vi "Editor Daten speichern (Sub.vi).vi"(0 "4":dbl[][](array[numeric]), 1 "Z 4":string, 2 "5":dbl[][](array[numeric]), 3 "Z 5":string, 4 "6":dbl[][](array[numeric]), 5 "Z 6":string, 6 "7":dbl[][](array[numeric]), 7 "Z 7":string, 8 "3":dbl[][](array[numeric]), 9 "8":dbl[][](array[numeric]), 10 "Z 3":string, 11 "Z 8":string, 12 "2":dbl[][](array[numeric]), 13 "9":dbl[][](array[numeric]), 14 "Z 2":string, 15 "Z 9":string, 16 "1":dbl[][](array[numeric]), 17 "10":dbl[][](array[numeric]), 18 "Z 1":string, 19 "Z 10":string, 21 "Formatierung+Namen":string="%d", 25 "Daten":string="%d", 26 "Modulname":string="%d") -> (23 "Ausgang":string)   [LabVIEW 2010]
panel:
  out "Verknüpfter String":string
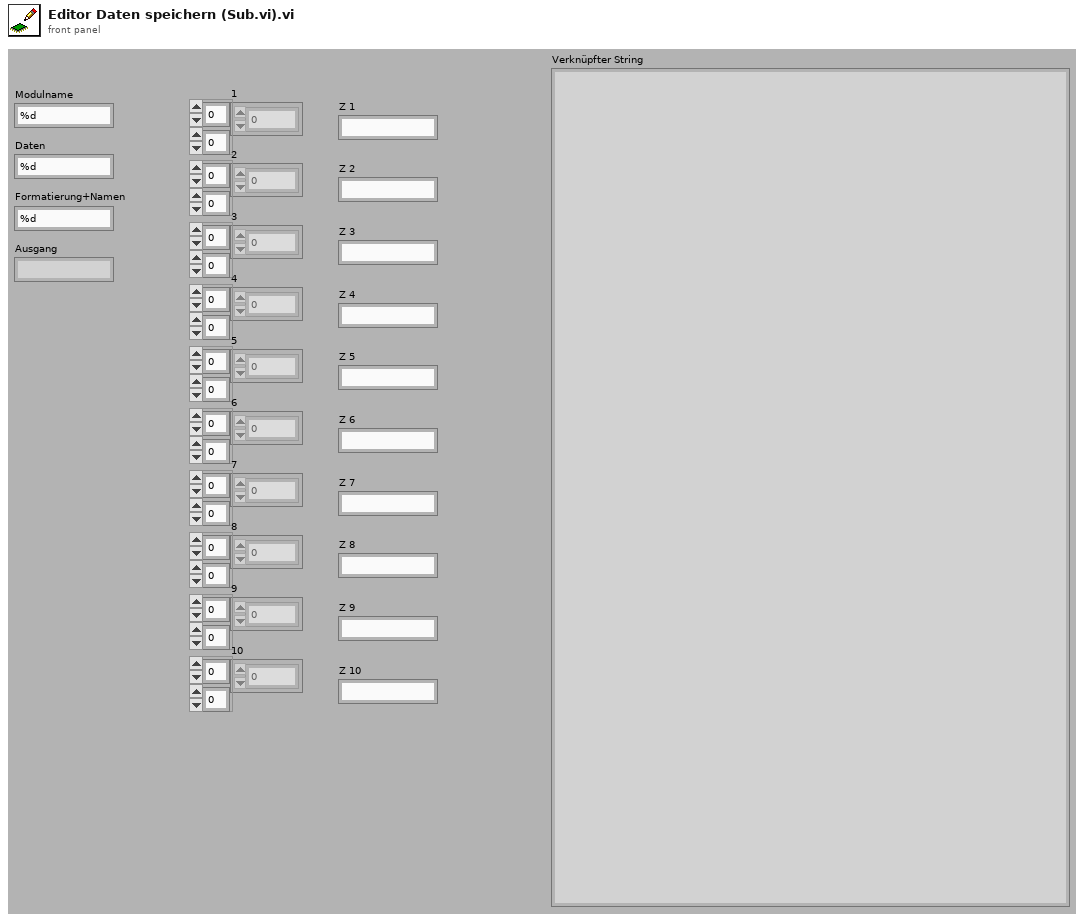
[diagram p1: front panel]
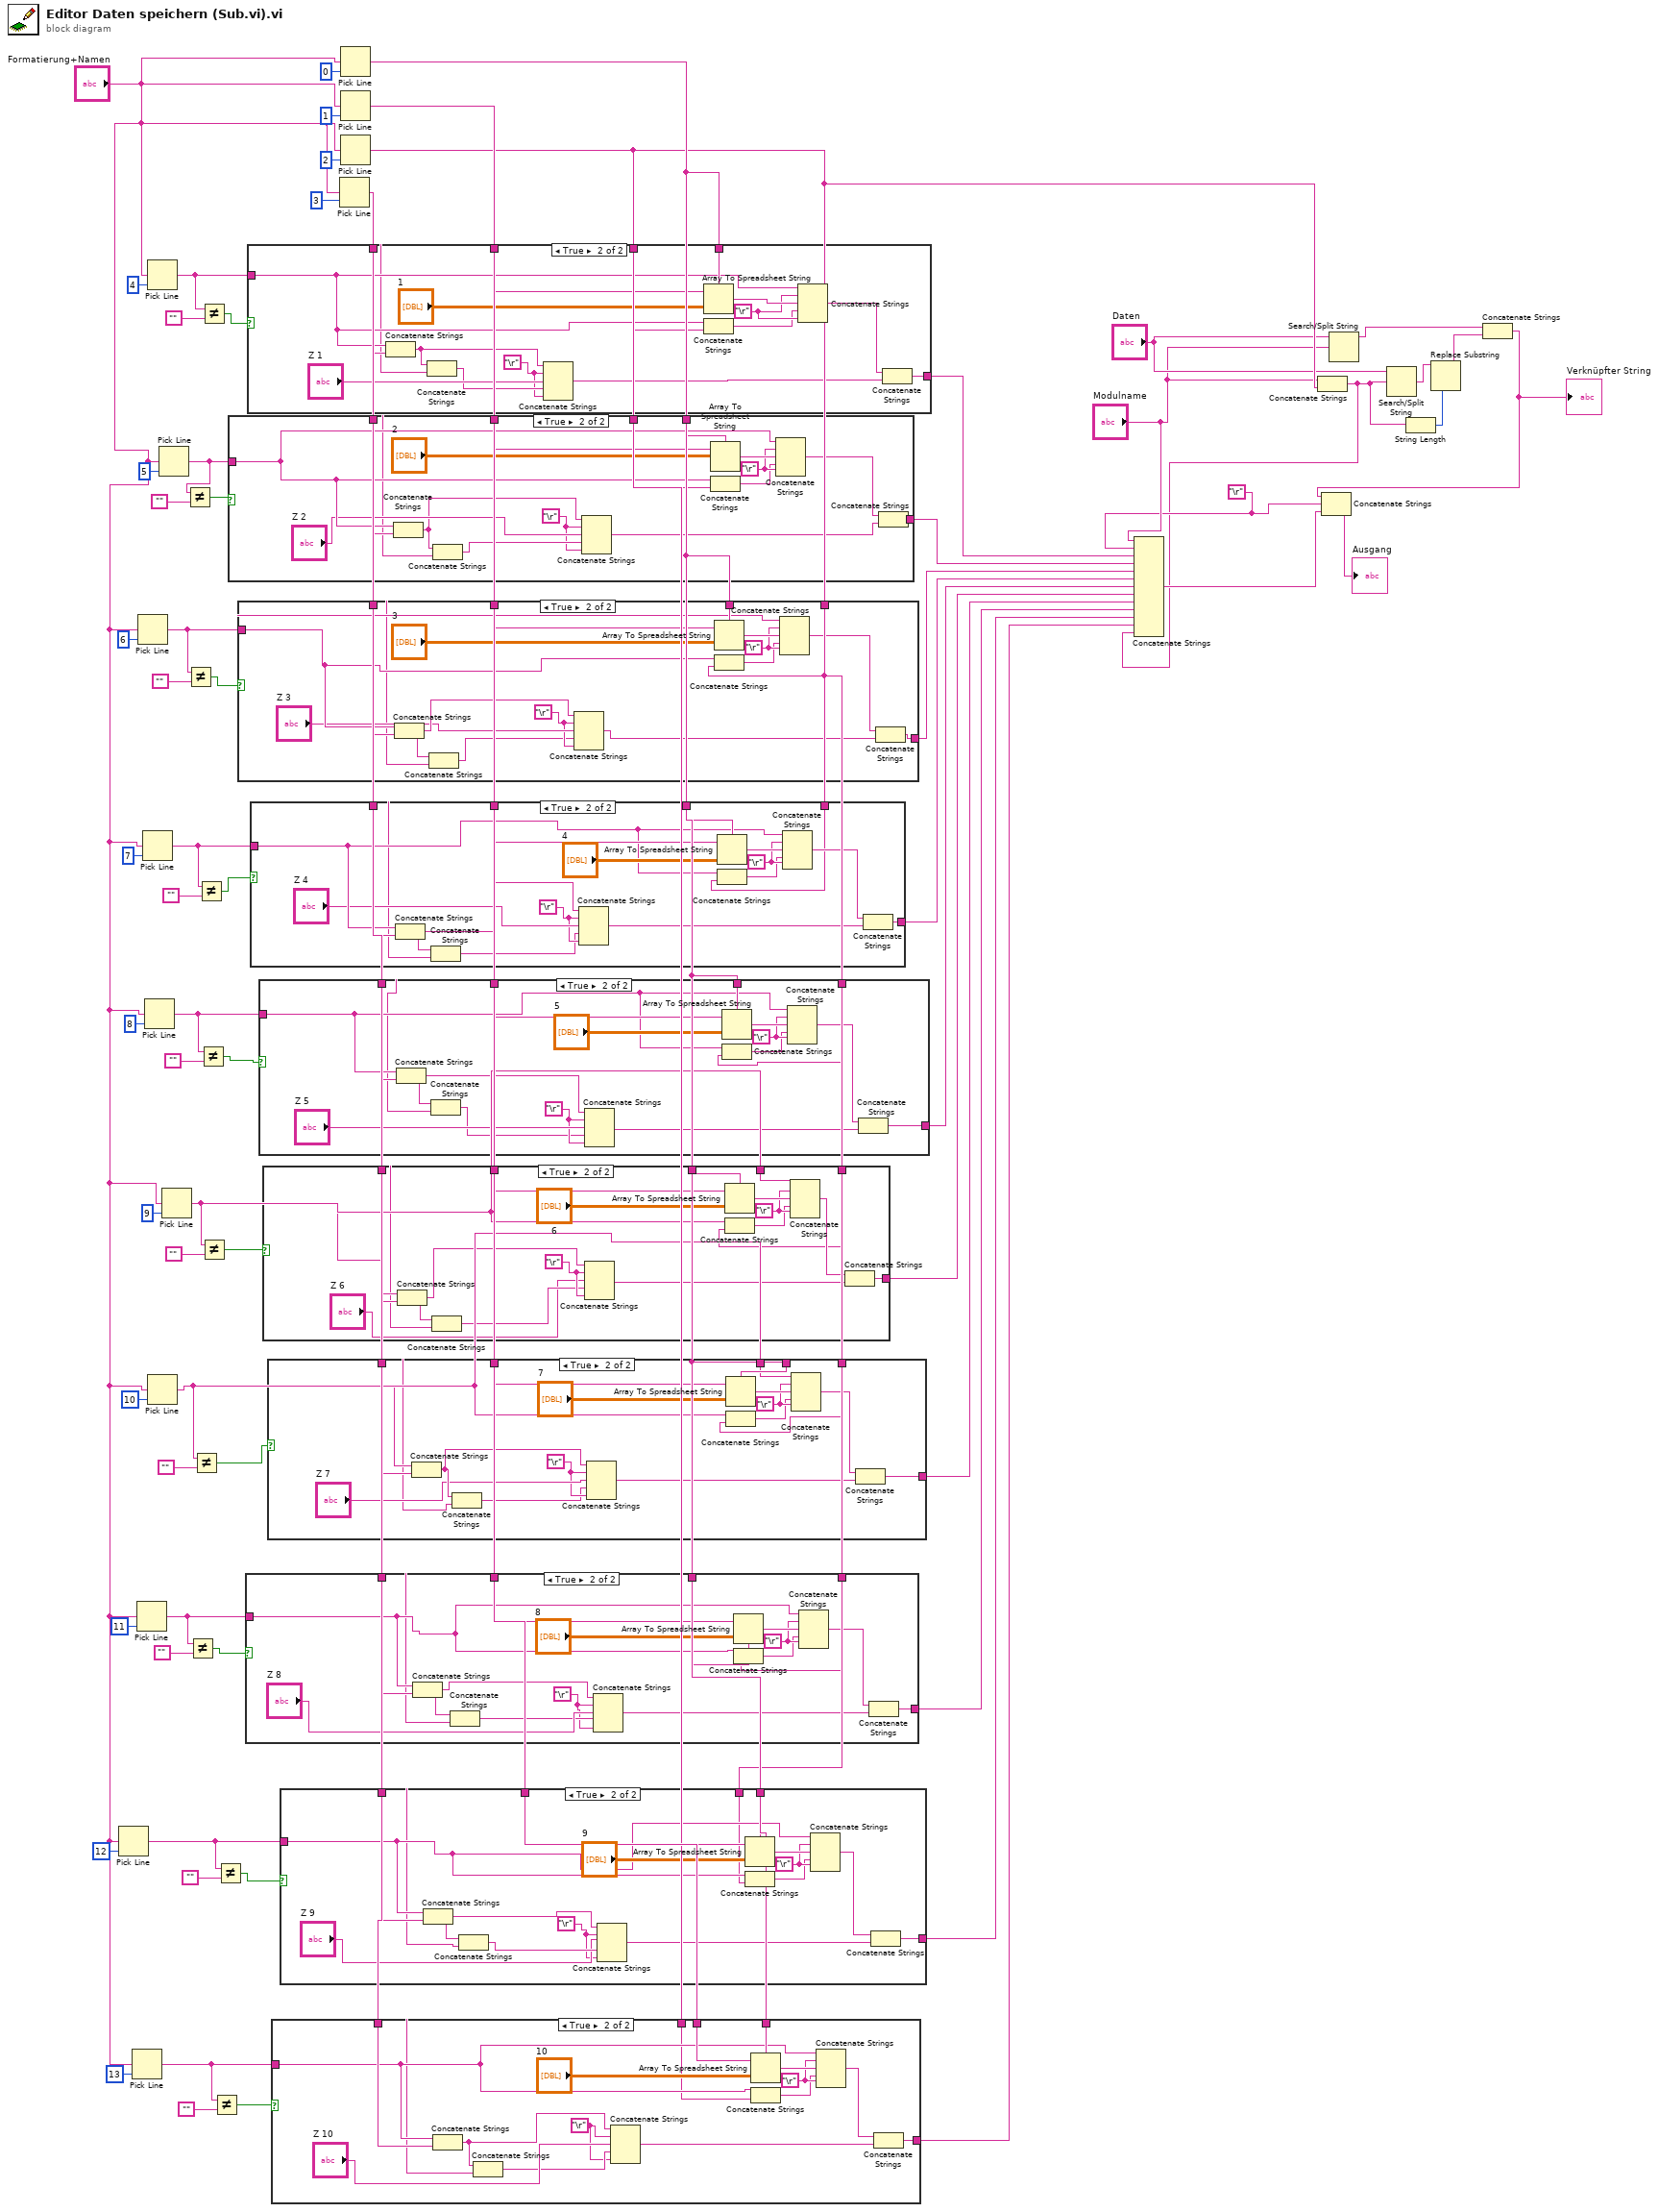
[diagram p0: block diagram]
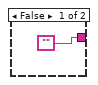
[diagram p2: hidden frame]
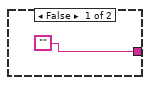
[diagram p3: hidden frame]
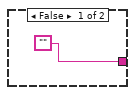
[diagram p4: hidden frame]
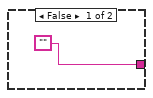
[diagram p5: hidden frame]
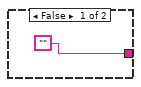
[diagram p6: hidden frame]
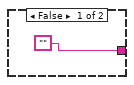
[diagram p7: hidden frame]
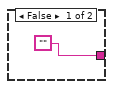
[diagram p8: hidden frame]
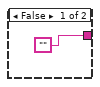
[diagram p9: hidden frame]
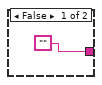
[diagram p10: hidden frame]
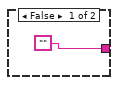
[diagram p11: hidden frame]
diagram:
  w32 = "\r"
  n1 = Pick Line(multi-line string="Formatierung+Namen", line index=12 ("Zeilenindex")) -> (output string=w15:string)  [unwired: 1 in]
  n2 = Pick Line(multi-line string="Formatierung+Namen", line index=13 ("Zeilenindex")) -> (output string=w17:string)  [unwired: 1 in]
  n3 = Pick Line(multi-line string="Formatierung+Namen", line index=11 ("Zeilenindex")) -> (output string=w13:string)  [unwired: 1 in]
  n4 = Pick Line(multi-line string="Formatierung+Namen", line index=6 ("Zeilenindex")) -> (output string=w3:string)  [unwired: 1 in]
  n5 = Pick Line(multi-line string="Formatierung+Namen", line index=7 ("Zeilenindex")) -> (output string=w6:string)  [unwired: 1 in]
  n6 = Pick Line(multi-line string="Formatierung+Namen", line index=8 ("Zeilenindex")) -> (output string=w7:string)  [unwired: 1 in]
  n7 = Pick Line(multi-line string="Formatierung+Namen", line index=4 ("Zeilenindex")) -> (output string=w29:string)  [unwired: 1 in]
  n8 = Pick Line(multi-line string="Formatierung+Namen", line index=10 ("Zeilenindex")) -> (output string=w11:string)  [unwired: 1 in]
  n9 = Pick Line(multi-line string="Formatierung+Namen", line index=5 ("Zeilenindex")) -> (output string=w1:string)  [unwired: 1 in]
  n10 = Pick Line(multi-line string="Formatierung+Namen", line index=9 ("Zeilenindex")) -> (output string=w9:string)  [unwired: 1 in]
  n11 = Not Equal?(x=w1, y="") -> (x != y?=w2:bool)
  n12 = Not Equal?(x=w3, y="") -> (x != y?=w4:bool)
  n13 = Not Equal?(x=w13, y="") -> (x != y?=w14:bool)
  n14 = Not Equal?(x=w11, y="") -> (x != y?=w12:bool)
  n15 = Not Equal?(x=w6, y="") -> (x != y?=w5:bool)
  n16 = Not Equal?(x=w7, y="") -> (x != y?=w8:bool)
  n17 = Not Equal?(x=w29, y="") -> (x != y?=w30:bool)
  n18 = Not Equal?(x=w9, y="") -> (x != y?=w10:bool)
  n19 = Not Equal?(x=w17, y="") -> (x != y?=w18:bool)
  n20 = Not Equal?(x=w15, y="") -> (x != y?=w16:bool)
  n21 = Pick Line(multi-line string="Formatierung+Namen", line index=3 ("Zeilenindex")) -> (output string=w53:string)  [unwired: 1 in]
  n22 = Pick Line(multi-line string="Formatierung+Namen", line index=0 ("Zeilenindex")) -> (output string=w66:string)  [unwired: 1 in]
  n23 = Pick Line(multi-line string="Formatierung+Namen", line index=1 ("Zeilenindex")) -> (output string=w67:string)  [unwired: 1 in]
  n24 = Pick Line(multi-line string="Formatierung+Namen", line index=2 ("Zeilenindex")) -> (output string=w42:string)  [unwired: 1 in]
  n25 = case shown="True" w2 {
    tunnel: w67 -> [_ w83]
    tunnel: w66 -> [_ w82]
    tunnel: w53 -> [_ w81]
    tunnel: w1 -> [_ w80]
    tunnel: ["" w75] -> w51
    tunnel: w42 -> [_ w72]
    frame False {
    }
    frame True {
      w73 = "\r"
      w86 = "\r"
      n26 = Concatenate Strings(w80, w81) -> (w78:string)
      n27 = Concatenate Strings(w78, w72) -> (w74:string)
      n28 = Concatenate Strings(w78, w73, "Z 2", w74, w73) -> (w76:string)
      n29 = Array To Spreadsheet String(delimiter (Tab)=w82, array="2", 3:w83) -> (spreadsheet string=w87:string)
      n30 = Concatenate Strings(w80, w72) -> (w85:string)
      n31 = Concatenate Strings(w80, w86, w87, w85, w86) -> (w77:string)
      n32 = Concatenate Strings(w77, w76) -> (w75:string)
    }
  }
  n33 = case shown="True" w4 {
    tunnel: w67 -> [_ w100]
    tunnel: w66 -> [_ w99]
    tunnel: w53 -> [_ w98]
    tunnel: w3 -> [_ w97]
    tunnel: ["" w92] -> w50
    tunnel: w42 -> [_ w89]
    frame False {
    }
    frame True {
      w91 = "\r"
      w103 = "\r"
      n34 = Concatenate Strings(w97, w98) -> (w96:string)
      n35 = Concatenate Strings(w96, w89) -> (w90:string)
      n36 = Concatenate Strings(w96, w91, "Z 3", w90, w91) -> (w93:string)
      n37 = Array To Spreadsheet String(delimiter (Tab)=w99, array="3", 3:w100) -> (spreadsheet string=w104:string)
      n38 = Concatenate Strings(w97, w89) -> (w102:string)
      n39 = Concatenate Strings(w97, w103, w104, w102, w103) -> (w94:string)
      n40 = Concatenate Strings(w94, w93) -> (w92:string)
    }
  }
  n41 = case shown="True" w14 {
    tunnel: w67 -> [_ w117]
    tunnel: w66 -> [_ w116]
    tunnel: w53 -> [_ w115]
    tunnel: w13 -> [_ w114]
    tunnel: ["" w109] -> w45
    tunnel: w42 -> [_ w106]
    frame False {
    }
    frame True {
      w107 = "\r"
      w120 = "\r"
      n42 = Concatenate Strings(w114, w115) -> (w113:string)
      n43 = Concatenate Strings(w113, w106) -> (w108:string)
      n44 = Concatenate Strings(w113, w107, "Z 8", w108, w107) -> (w110:string)
      n45 = Array To Spreadsheet String(delimiter (Tab)=w116, array="8", 3:w117) -> (spreadsheet string=w121:string)
      n46 = Concatenate Strings(w114, w106) -> (w119:string)
      n47 = Concatenate Strings(w114, w120, w121, w119, w120) -> (w111:string)
      n48 = Concatenate Strings(w111, w110) -> (w109:string)
    }
  }
  n49 = case shown="True" w30 {
    tunnel: w67 -> [_ w134]
    tunnel: w66 -> [_ w133]
    tunnel: w53 -> [_ w132]
    tunnel: w29 -> [_ w131]
    tunnel: ["" w126] -> w52
    tunnel: w42 -> [_ w123]
    frame False {
    }
    frame True {
      w124 = "\r"
      w137 = "\r"
      n50 = Concatenate Strings(w131, w132) -> (w130:string)
      n51 = Concatenate Strings(w130, w123) -> (w125:string)
      n52 = Concatenate Strings(w130, w124, "Z 1", w125, w124) -> (w127:string)
      n53 = Array To Spreadsheet String(delimiter (Tab)=w133, array="1", 3:w134) -> (spreadsheet string=w138:string)
      n54 = Concatenate Strings(w131, w123) -> (w136:string)
      n55 = Concatenate Strings(w131, w137, w138, w136, w137) -> (w128:string)
      n56 = Concatenate Strings(w128, w127) -> (w126:string)
    }
  }
  n57 = case shown="True" w5 {
    tunnel: w67 -> [_ w151]
    tunnel: w66 -> [_ w150]
    tunnel: w53 -> [_ w149]
    tunnel: w6 -> [_ w148]
    tunnel: ["" w143] -> w49
    tunnel: w42 -> [_ w140]
    frame False {
    }
    frame True {
      w142 = "\r"
      w154 = "\r"
      n58 = Concatenate Strings(w148, w149) -> (w147:string)
      n59 = Concatenate Strings(w147, w140) -> (w141:string)
      n60 = Concatenate Strings(w147, w142, "Z 4", w141, w142) -> (w144:string)
      n61 = Array To Spreadsheet String(delimiter (Tab)=w150, array="4", 3:w151) -> (spreadsheet string=w155:string)
      n62 = Concatenate Strings(w148, w140) -> (w153:string)
      n63 = Concatenate Strings(w148, w154, w155, w153, w154) -> (w145:string)
      n64 = Concatenate Strings(w145, w144) -> (w143:string)
    }
  }
  n65 = case shown="True" w8 {
    tunnel: w67 -> [_ w168]
    tunnel: w66 -> [_ w167]
    tunnel: w53 -> [_ w166]
    tunnel: w7 -> [_ w165]
    tunnel: ["" w160] -> w48
    tunnel: w42 -> [_ w157]
    frame False {
    }
    frame True {
      w159 = "\r"
      w171 = "\r"
      n66 = Concatenate Strings(w165, w166) -> (w164:string)
      n67 = Concatenate Strings(w164, w157) -> (w158:string)
      n68 = Concatenate Strings(w164, w159, "Z 5", w158, w159) -> (w161:string)
      n69 = Array To Spreadsheet String(delimiter (Tab)=w167, array="5", 3:w168) -> (spreadsheet string=w172:string)
      n70 = Concatenate Strings(w165, w157) -> (w170:string)
      n71 = Concatenate Strings(w165, w171, w172, w170, w171) -> (w162:string)
      n72 = Concatenate Strings(w162, w161) -> (w160:string)
    }
  }
  n73 = case shown="True" w10 {
    tunnel: w67 -> [_ w185]
    tunnel: w66 -> [_ w184]
    tunnel: w53 -> [_ w183]
    tunnel: w9 -> [_ w182]
    tunnel: ["" w178] -> w47
    tunnel: w42 -> [_ w174]
    frame False {
    }
    frame True {
      w177 = "\r"
      w188 = "\r"
      n74 = Concatenate Strings(w182, w183) -> (w181:string)
      n75 = Concatenate Strings(w181, w174) -> (w176:string)
      n76 = Concatenate Strings(w181, w177, "Z 6", w176, w177) -> (w179:string)
      n77 = Array To Spreadsheet String(delimiter (Tab)=w184, array="6", 3:w185) -> (spreadsheet string=w189:string)
      n78 = Concatenate Strings(w182, w174) -> (w187:string)
      n79 = Concatenate Strings(w182, w188, w189, w187, w188) -> (w180:string)
      n80 = Concatenate Strings(w180, w179) -> (w178:string)
    }
  }
  n81 = case shown="True" w12 {
    tunnel: w67 -> [_ w202]
    tunnel: w66 -> [_ w201]
    tunnel: w53 -> [_ w200]
    tunnel: w11 -> [_ w199]
    tunnel: ["" w194] -> w46
    tunnel: w42 -> [_ w191]
    frame False {
    }
    frame True {
      w193 = "\r"
      w205 = "\r"
      n82 = Concatenate Strings(w199, w200) -> (w198:string)
      n83 = Concatenate Strings(w198, w191) -> (w192:string)
      n84 = Concatenate Strings(w198, w193, "Z 7", w192, w193) -> (w195:string)
      n85 = Array To Spreadsheet String(delimiter (Tab)=w201, array="7", 3:w202) -> (spreadsheet string=w206:string)
      n86 = Concatenate Strings(w199, w191) -> (w204:string)
      n87 = Concatenate Strings(w199, w205, w206, w204, w205) -> (w196:string)
      n88 = Concatenate Strings(w196, w195) -> (w194:string)
    }
  }
  n89 = case shown="True" w18 {
    tunnel: w67 -> [_ w219]
    tunnel: w66 -> [_ w218]
    tunnel: w53 -> [_ w217]
    tunnel: w17 -> [_ w216]
    tunnel: ["" w211] -> w43
    tunnel: w42 -> [_ w209]
    frame False {
    }
    frame True {
      w208 = "\r"
      w222 = "\r"
      n90 = Concatenate Strings(w216, w217) -> (w215:string)
      n91 = Concatenate Strings(w215, w209) -> (w210:string)
      n92 = Concatenate Strings(w215, w208, "Z 10", w210, w208) -> (w212:string)
      n93 = Array To Spreadsheet String(delimiter (Tab)=w218, array="10", 3:w219) -> (spreadsheet string=w223:string)
      n94 = Concatenate Strings(w216, w209) -> (w221:string)
      n95 = Concatenate Strings(w216, w222, w223, w221, w222) -> (w213:string)
      n96 = Concatenate Strings(w213, w212) -> (w211:string)
    }
  }
  n97 = case shown="True" w16 {
    tunnel: w67 -> [_ w236]
    tunnel: w66 -> [_ w235]
    tunnel: w53 -> [_ w234]
    tunnel: w15 -> [_ w233]
    tunnel: ["" w229] -> w44
    tunnel: w42 -> [_ w225]
    frame False {
    }
    frame True {
      w226 = "\r"
      w239 = "\r"
      n98 = Concatenate Strings(w233, w234) -> (w232:string)
      n99 = Concatenate Strings(w232, w225) -> (w228:string)
      n100 = Concatenate Strings(w232, w226, "Z 9", w228, w226) -> (w230:string)
      n101 = Array To Spreadsheet String(delimiter (Tab)=w235, array="9", 3:w236) -> (spreadsheet string=w240:string)
      n102 = Concatenate Strings(w233, w225) -> (w238:string)
      n103 = Concatenate Strings(w233, w239, w240, w238, w239) -> (w231:string)
      n104 = Concatenate Strings(w231, w230) -> (w229:string)
    }
  }
  n105 = Concatenate Strings("Modulname", w42) -> (w31:string)
  n106 = Concatenate Strings("Modulname", w32, w52, w51, w50, w49, w48, w47, w46, w45, w44, w43, w31) -> (w35:string)
  n107 = Search/Split String(string="Daten", search string/char (-)="Modulname") -> (substring before match=w41:string)  [unwired: 1 in, 2 out]
  n108 = Search/Split String(string="Daten", search string/char (-)=w31) -> (match + rest of string=w38:string)  [unwired: 1 in, 2 out]
  n109 = String Length(string=w31) -> (length=w39:i32)
  n110 = Replace Substring(2:w39, 5:w38) -> (1:w37:string)  [unwired: 2 in, 1 out]
  n111 = Concatenate Strings(w41, w37) -> (w34:string)
  "Verknüpfter String" <- w34
  n112 = Concatenate Strings(w34, w32, w35) -> (→"Ausgang":string)
